vi "PYTHON Close Session__ogtk.vi"(4 "error in (no error)":errorcluster, 7 "Python Session in":T1) -> (0 "error out":errorcluster)   [LabVIEW 2014]
doc: "Closes a Python script session and disposes of any resources assigned to this session."
uses:
  <userlib>/_OpenG.lib/labpython/labpython.llb/PYTHON Session Refnum__ogtk.ctl
  <userlib>/_OpenG.lib/labpython/lvpython.dll
panel:
  # "PYTHON Close Session.vi\n\nClose the session context and dispose of any related resources\n\nCopyright (C) 2002 Rolf Kalbermatter rolf.kalbermatter@citeng.com\nCopyright (C) 2002 James Kring jim@jimkring.com\n\nPlease visit http://www.OpenG.org to learn about the\nOpen Source LabVIEW software movement.\n\nThis library is free software; you can redistribute it and/or\nmodify it under the terms of the GNU Lesser General Public\nLicense as published by the Free Software Foundation; either\nversion 2.1 of the License, or (at your option) any later version.\nThis library is distributed in the hope that it will be useful,\nbut WITHOUT ANY WARRANTY; without even the implied warranty of\nMERCHANTABILITY or FITNESS FOR A PARTICULAR PURPOSE. See the GNU\nLesser General Public License for more details.\nYou should have received a copy of the GNU Lesser General Public\nLicense along with this library; if not, write to the Free Software\nFoundation, Inc., 59 Temple Place, Suite 330, Boston, MA 02111-1307 USA"
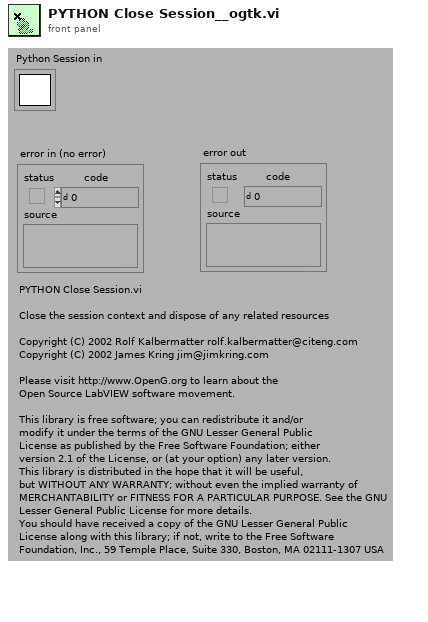
[diagram p1: front panel]
types:
  T1 = typedef "PYTHON Session Refnum__ogtk.ctl" = refnum<k1>
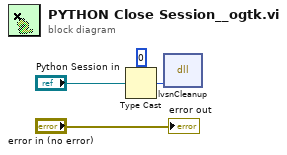
[diagram p0: block diagram]
diagram:
  n1 = Type Cast(type=u32 0 ("session"), x="Python Session in") -> (*(type *) &x=w2:u32)
  n2 = dll-call lib="C:/Program Files (x86)/National Instruments/LabVIEW 2014/user.lib/_OpenG.lib/labpython/lvpython.*" fn="lvsnCleanup"("session"=w2) -> ()  [unwired: 5 in, 2 out]
  "error out" <- "error in (no error)"
